vi "Get Scanner (continuous).vi"(8 "error in (no error)":errorcluster, 11 "Varian Magnet.lvclass":refnum<class "Varian Magnet.lvclass">) -> (0 "error out":errorcluster, 3 "Default Scanner out":refnum<class "Scanner.lvclass">)   [LabVIEW 2012, in "Varian Magnet.lvclass"]
uses:
  Varian Magnet.lvclass
  Scanners/Scanner/Scanner.lvclass
  Scanners/Varian Magnet Scan/Varian Continuous/Varian Continuous.lvclass
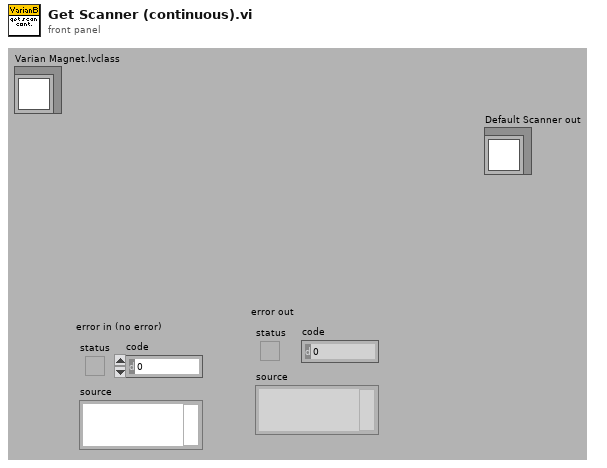
[diagram p1: front panel]
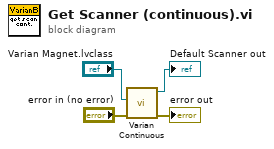
[diagram p0: block diagram]
diagram:
  n1 = call "Varian Continuous.vi"("error in"="error in (no error)", "Varian Magnet.lvclass"="Varian Magnet.lvclass") -> ("error out"=→"error out":errorcluster, "Varian Continous out"=→"Default Scanner out":refnum<class "Varian Continuous.lvclass">)  [unwired: 8 in]
